vi "Update-characteristics-chart.vi"(8 "error in":errorcluster, 10 "Data ref. in":refnum<data-value>, 11 "UI ref. in":refnum<data-value>) -> (0 "error IO":errorcluster, 2 "Data ref.":refnum<data-value>, 3 "UI ref.":refnum<data-value>)   [LabVIEW 2013, in "CameraVision.lvlib" / "CV-UI.lvclass"]
doc: "This function collects image and melt pool characteristics data from the image processing routine. The last 1000 data points for each active camera are displayed in a sweep chart.\nThis function is considered low priority. The availability of new data is communicated through a notifier, which can lead to data loss if the system is slowed down.\nThis function is active independent of the 'Image refresh' button value."
uses:
  CV-UI.lvclass
  Main/CV-Main.lvclass
  Display-names.ctl
  Main/CV-Main.lvclass/CV-Main.ctl
  CV-UI.lvclass/CV-UI.ctl
  Read Display refs.vi
  Main/Read Processing.vi
  Main/Read UI buffer.vi
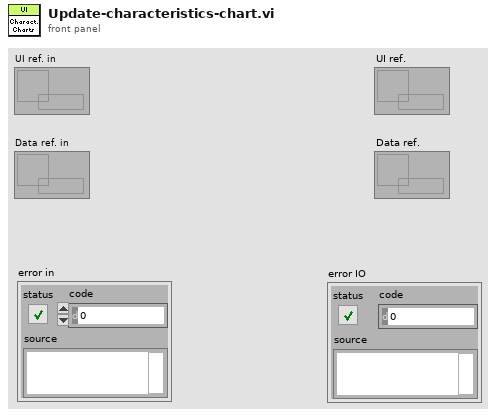
[diagram p1: front panel]
types:
  T1 = typedef "CameraVision.lvlib/CV-UI.lvclass/Display-names.ctl" = enum16{"State", "Action", "Current image", "Framerate", "Frametime", "Process buffer", "Storage buffer", "Free disk space", "Total disk space", "Information", "Histogram", "Camera 1", "Camera 2", "Camera 1 chart", "Camera 2 chart", "Browser", "Temperature", "Map", "Status overview", "Characteristics", "Temper characteristics"}
  T2 = typedef "CameraVision.lvlib/Buffers.lvclass/Storage-buffer.ctl" = cluster{"Index":i32, "Time":timestamp, "Raw images":T3[], "Corrected images":T3[], "Binary images":T3[], "Temperature characteristics":T4, "Characteristics":T5[], "Temperature field":dbl[][]}
  T3 = typedef "IMAQ Image.ctl" = refnum<image>
  T4 = typedef "CameraVision.lvlib/Temperature.lvclass/Temperature-characteristics.ctl" = cluster{"Average temperature ":dbl, "Max. temperature":dbl, "Min. temperature":dbl, "Stand. dev. temperature":dbl, "Datapoints":dbl}
  T5 = typedef "CameraVision.lvlib/Analysis.lvclass/Characteristics-cluster.ctl" = cluster{"Average intensity":dbl, "Peak intensity":dbl, "Melt-pool size":dbl, "Melt-pool aspect ratio":dbl, "Melt-pool fragments":dbl, "Centre of mass X":dbl, "Centre of mass Y":dbl, "Orientation":dbl}
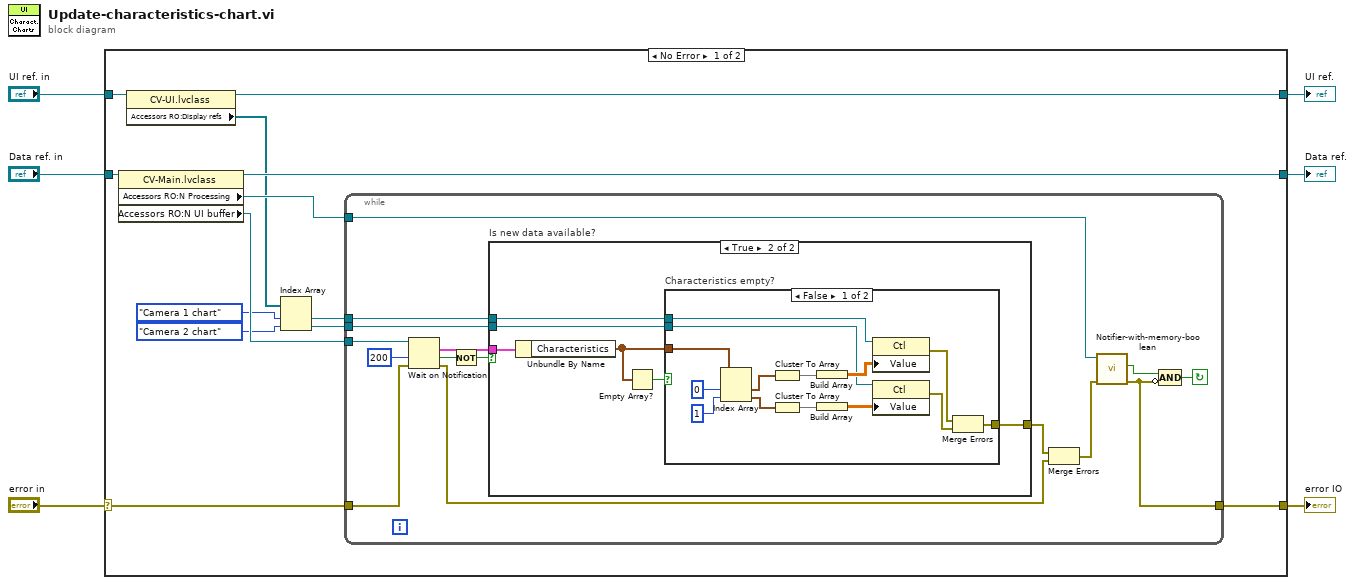
[diagram p0: block diagram]
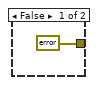
[diagram p2: hidden frame]
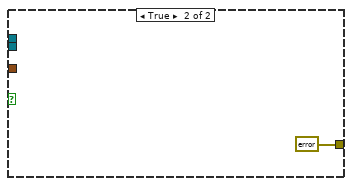
[diagram p3: hidden frame]
diagram:
  n1 = case shown="No Error" "error in" {
    selector: "error in" -> [w14 w59]
    tunnel: [w19 w59] -> w6
    tunnel: "UI ref. in" -> [w18 w58]
    tunnel: "Data ref. in" -> [w17 w57]
    tunnel: [w16 w57] -> w1
    tunnel: [w15 w58] -> w2
    frame No Error {
      n2 = property class="CV-Main.lvclass"(reference=w17) -> (reference out=w16:refnum<data-value>, "Accessors RO:N Processing"=w13:refnum<notifier>, "Accessors RO:N UI buffer"=w12:refnum<notifier>)  [unwired: 1 in, 1 out]
      n3 = property class="CV-UI.lvclass"(reference=w18) -> (reference out=w15:refnum<data-value>, "Accessors RO:Display refs"=w11:refnum<vi>[])  [unwired: 1 in, 1 out]
      n4 = Index Array(array=w11, index #1=Display-names."Camera 1 chart" ("Dislay"), index #2=Display-names."Camera 2 chart" ("Dislay")) -> (element #1=w7:refnum<vi>, element #2=w8:refnum<vi>)
      n5 = while {
        tunnel: w14 -> [w25]
        tunnel: [w21] -> w19
        tunnel: w13 -> [w32]
        tunnel: w12 -> [w31]
        tunnel: w7 -> [w27]
        tunnel: w8 -> [w26]
        stop <- w33 continue-if-true
        n6 = Wait on Notification(notifier=w31, timeout in ms (-1)=200, error in (no error)=w25) -> (notification=w28:T2, timed out?=w30:bool, error out=w23:errorcluster)  [unwired: 1 in, 1 out]
        n7 = Not(x=w30) -> (.not. x?=w29:bool)
        n8 = case "Is new data available?" shown="True" w29 {
          tunnel: w27 -> [_ w41]
          tunnel: w26 -> [_ w40]
          tunnel: [errorcluster {"status"=FALSE, "code"=0, "source"=""} ("error IO") w36] -> w24
          tunnel: w28 -> [_ w38]
          frame False {
          }
          frame True {
            n9 = Unbundle By Name(w38) -> ("Characteristics"=w37:T5[])
            n10 = Empty Array?(array=w37) -> (empty?=w39:bool)
            n11 = case "Characteristics empty?" shown="False" w39 {
              tunnel: w41 -> [w49 _]
              tunnel: w40 -> [w47 _]
              tunnel: w37 -> [w45 _]
              tunnel: [w42 errorcluster {"status"=FALSE, "code"=0, "source"=""} ("error IO")] -> w36
              frame False {
                n12 = Index Array(array=w45, index #1=0 ("index (page)"), index #2=1 ("index (page)")) -> (element #1=w53:T5, element #2=w50:T5)
                n13 = Cluster To Array(cluster=w53) -> (array=w52:dbl[])
                n14 = Cluster To Array(cluster=w50) -> (array=w51:dbl[])
                n15 = Build Array(w52) -> (w48:dbl[][])
                n16 = Build Array(w51) -> (w46:dbl[][])
                n17 = property class="Ctl"(reference=w49, "Value"=w48) -> (error out=w44:errorcluster)  [unwired: 1 in, 1 out]
                n18 = property class="Ctl"(reference=w47, "Value"=w46) -> (error out=w43:errorcluster)  [unwired: 1 in, 1 out]
                n19 = Merge Errors(w44, w43) -> (w42:errorcluster)
              }
              frame True {
              }
            }
          }
        }
        n20 = Merge Errors(w24, w23) -> (w22:errorcluster)
        n21 = call "Notifier-with-memory-boolean.vi"("error in"=w22, "Notifier in"=w32) -> ("error IO"=w21:errorcluster, "Notification"=w34:bool)  [unwired: 8 in]
        n22 = Compound Arithmetic op=AND(w34, invert w21) -> (w33:bool)
      }
    }
    frame Error {
    }
  }
  "error IO" <- w6
  "UI ref." <- w2
  "Data ref." <- w1
